vi "Configure DC Current.vi"(4 "Set Aperture or NPLC? (T: Aperture)":bool, 6 "NPLC":dbl=1.0 min=0.0005 max=15.0 step=1.0, 7 "Aperture Seconds":dbl=0.01616 min=8.333e-06 max=0.25 step=1e-06, 8 "error in (no error)":errorcluster, 9 "Manual Range":dbl=3.0 min=-3.0 max=3.0, 10 "Auto Range? (T: Auto)":bool, 11 "VISA resource name":refnum<visa-resource-name>) -> (0 "error out":errorcluster, 3 "VISA resource name out":refnum<visa-resource-name>)   [LabVIEW 2018, in "Keithley DMM7512.lvlib"]
doc: "This VI configures the DC Current measurement and the related parameters."
uses:
  <instrlib>/Keithley DMM7512/Keithley DMM7512.lvlib
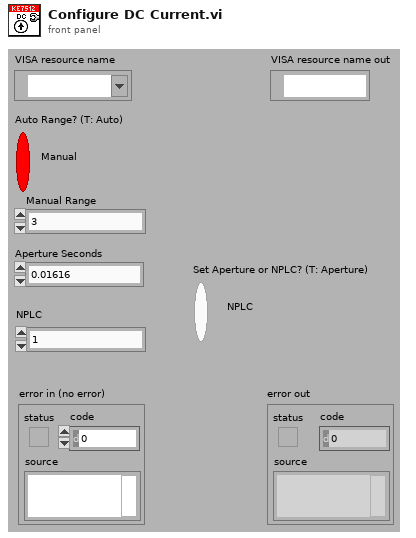
[diagram p1: front panel]
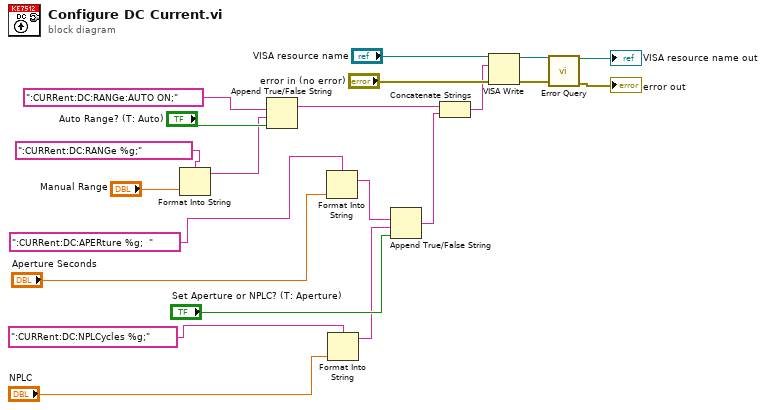
[diagram p0: block diagram]
diagram:
  n1 = Format Into String(format string=":CURRent:DC:RANGe %g;", "Manual Range") -> (resulting string=w15:string)  [unwired: 2 in, 1 out]
  n2 = Append True/False String(1:"Auto Range? (T: Auto)", 2:w15, 3:":CURRent:DC:RANGe:AUTO ON;") -> (0:w1:string)  [unwired: 1 in]
  n3 = Format Into String(format string=":CURRent:DC:APERture %g;  ", "Aperture Seconds") -> (resulting string=w5:string)  [unwired: 2 in, 1 out]
  n4 = Format Into String(format string=":CURRent:DC:NPLCycles %g;", "NPLC") -> (resulting string=w3:string)  [unwired: 2 in, 1 out]
  n5 = Append True/False String(1:"Set Aperture or NPLC? (T: Aperture)", 2:w3, 3:w5) -> (0:w2:string)  [unwired: 1 in]
  n6 = Concatenate Strings(w1, w2) -> (w12:string)
  n7 = VISA Write(VISA resource name="VISA resource name", write buffer=w12, error in (no error)="error in (no error)") -> (VISA resource name out=w11:refnum<visa-resource-name>, error out=w10:errorcluster)  [unwired: 1 out]
  n8 = call <instrlib>:"Error Query.vi"("error in (no error)"=w10, "VISA resource name"=w11) -> ("error out"=→"error out":errorcluster, "VISA resource name out"=→"VISA resource name out":refnum<visa-resource-name>)  [unwired: 6 in, 2 out]
